vi "Handle Message.vi"(8 "error in (no error)":errorcluster, 9 "Message Completion Handler":refnum<class "Message Completion Handler.lvclass">, 10 "Message":string, 11 "RandomNumberLogger in":refnum<class "RandomNumberLogger.lvclass">) -> (0 "error out":errorcluster, 1 "Synchronously Complete Message?":bool=TRUE, 2 "Message Response":string, 3 "RandomNumberLogger out":refnum<class "RandomNumberLogger.lvclass">)   [LabVIEW 2020, in "RandomNumberLogger.lvlib" / "RandomNumberLogger.lvclass"]
doc: "<b>Handle Message</b>\nThis method allows you to handle messages received from other plugins/services. If you don't put handlers here for messages, then all messages broadcast to plugins will be thrown away by this plugin. If you need to handle a specific message (like pause, resume, etc.) the handler needs to be written here."
uses:
  RandomNumberLogger.lvclass
  RandomNumberLogger.lvclass/RandomNumberLogger.ctl
  <vilib>/ADAS Record/Utilities/TypeDefs/ADAS gRPC/DataStreamGrpc Message.ctl
  <vilib>/ADAS Record/Utilities/ADAS Utilities.lvlib
  <vilib>/FlexLogger/SDK/PluginSDK.lvlibp/PEFClasses/SDK/Message Completion Handler/Message Completion Handler.lvclass
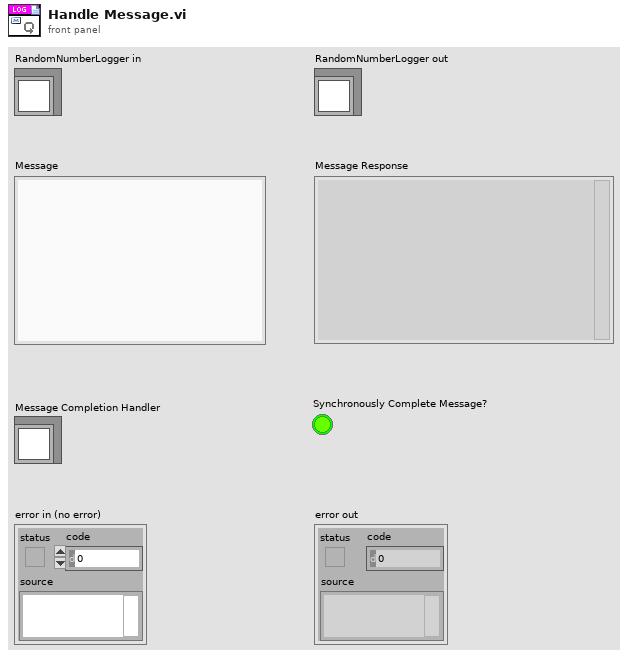
[diagram p1: front panel]
types:
  T1 = typedef "ADAS Utilities.lvlib/DataStreamGrpc Message.ctl" = cluster{"messageName":string, "details":string}
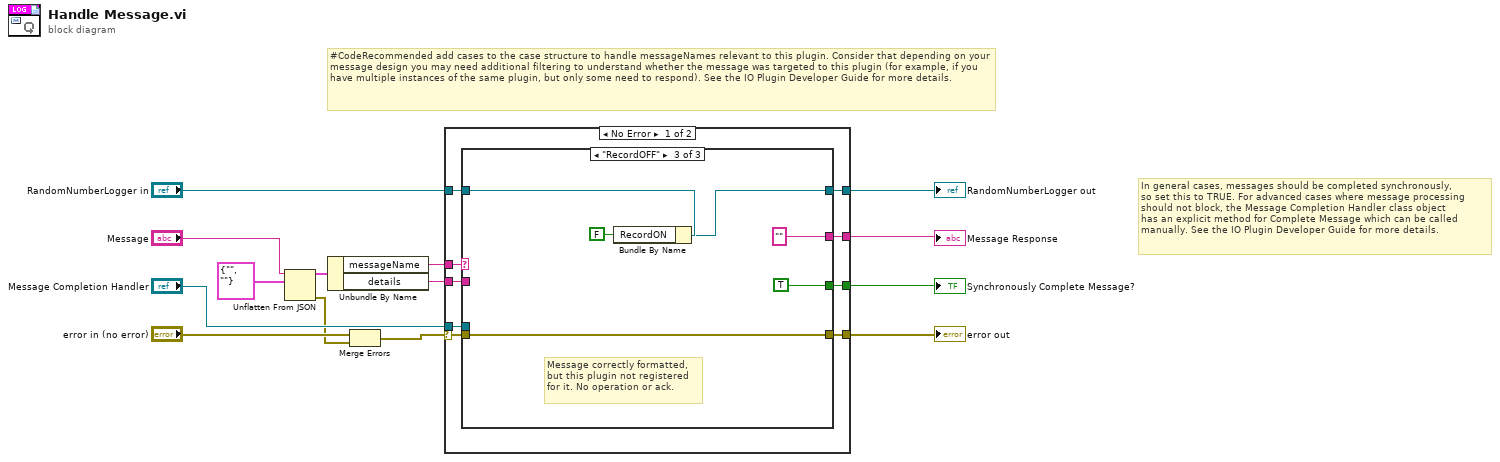
[diagram p0: block diagram]
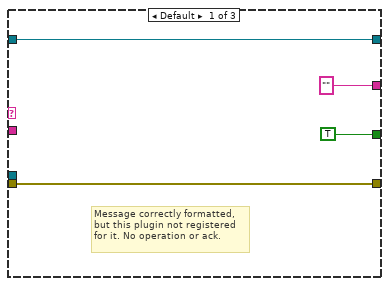
[diagram p2: hidden frame]
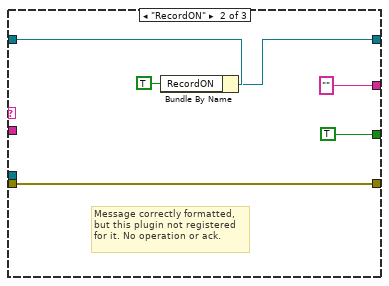
[diagram p3: hidden frame]
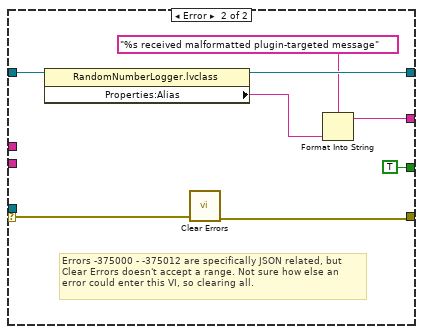
[diagram p4: hidden frame]
diagram:
  # "In general cases, messages should be completed synchronously,\nso set this to TRUE. For advanced cases where message processing\nshould not block, the Message Completion Handler class object\nhas an explicit method for Complete Message which can be called\nmanually. See the IO Plugin Developer Guide for more details."
  # "#CodeRecommended add cases to the case structure to handle messageNames relevant to this plugin. Consider that depending on your message design you may need additional filtering to understand whether the message was targeted to this plugin (for example, if you have multiple instances of the same plugin, but only some need to respond). See the IO Plugin Developer Guide for more details."
  n1 = Unflatten From JSON(JSON string="Message", type and defaults=T1 {"messageName"="", "details"=""} ("DataStreamGrpc Message")) -> (value=w7:T1, error out=w1:errorcluster)  [unwired: 5 in]
  n2 = Unbundle By Name(w7) -> ("messageName"=w6:string, "details"=w5:string)
  n3 = Merge Errors("error in (no error)", w1) -> (w2:errorcluster)
  n4 = case shown="No Error" w2 {
    selector: w2 -> [w15 w47]
    tunnel: [w23 w46] -> w14
    tunnel: [w22 w43] -> w13
    tunnel: "Message Completion Handler" -> [w21 _]
    tunnel: "RandomNumberLogger in" -> [w20 w44]
    tunnel: w6 -> [w19 _]
    tunnel: w5 -> [w18 _]
    tunnel: [w17 w40] -> w4
    tunnel: [w16 TRUE ("Synchronously Complete Message?")] -> w3
    frame No Error {
      n5 = case shown="\"RecordOFF\"" w19 {
        tunnel: [w27 w33 w39] -> w23
        tunnel: [w26 w29 w35] -> w22
        tunnel: w15 -> [w27 w33 w39]
        tunnel: w21 -> [_ _ _]
        tunnel: w20 -> [w26 w30 w36]
        tunnel: w18 -> [_ _ _]
        tunnel: ["" ("Message Response") "" ("Message Response") "" ("Message Response")] -> w17
        tunnel: [TRUE ("Synchronously Complete Message?") TRUE ("Synchronously Complete Message?") TRUE ("Synchronously Complete Message?")] -> w16
        frame Default {
          # "Message correctly formatted,\nbut this plugin not registered\nfor it. No operation or ack."
        }
        frame "RecordON" {
          # "Message correctly formatted,\nbut this plugin not registered\nfor it. No operation or ack."
          n6 = Bundle By Name(cluster=w30, "RecordON"=TRUE) -> (w29:refnum<class "RandomNumberLogger.lvclass">)
        }
        frame "RecordOFF" {
          # "Message correctly formatted,\nbut this plugin not registered\nfor it. No operation or ack."
          n7 = Bundle By Name(cluster=w36, "RecordON"=FALSE) -> (w35:refnum<class "RandomNumberLogger.lvclass">)
        }
      }
    }
    frame Error {
      # "Errors -375000 - -375012 are specifically JSON related, but \nClear Errors doesn't accept a range. Not sure how else an \nerror could enter this VI, so clearing all."
      n8 = property class="RandomNumberLogger.lvclass"(reference=w44) -> (reference out=w43:refnum<class "RandomNumberLogger.lvclass">, "Properties:Alias"=w41:string)  [unwired: 1 in, 1 out]
      n9 = call <vilib>:"Clear Errors.vi"("error in (no error)"=w47) -> ("error out"=w46:errorcluster)  [unwired: 5 in, 1 out]
      n10 = Format Into String(format string="%s received malformatted plugin-targeted message", w41) -> (resulting string=w40:string)  [unwired: 2 in, 1 out]
    }
  }
  "error out" <- w14
  "RandomNumberLogger out" <- w13
  "Message Response" <- w4
  "Synchronously Complete Message?" <- w3
